vi "Test System.vi"() -> ()   [LabVIEW 2015]
uses:
  CAN Communication/Gas/Typedefs/Valves.ctl
  CAN Communication/Peltier/Typedefs/Peltier Temperature Sensors.ctl
  CAN Communication/Gas/Gas.lvclass
  Common/Buffers/Snapshot/Snapshot.lvclass
  CAN Communication/Peltier/Peltier.lvclass
panel:
  out "Status":string
  out "Temp":dbl caption="H2 Temp C" format="%#.2g"
  out "PPM":dbl caption="H2 PPM" format="%#.2g"
  in  "H2":bool
  out "Gas Board Errors":errorcluster
  out "Oil Present?":string
  in  "Oil Pres":bool
  out "Pelt":errorcluster caption="Peltier Board Errors"
  out "TS5":dbl caption="Temp Sensor 5" format="%#.2g"
  out "TS4":dbl caption="Temp Sensor 4" format="%#.2g"
  out "TS3":dbl caption="Temp Sensor 3" format="%#.2g"
  out "TS2":dbl caption="Temp Sensor 2" format="%#.2g"
  out "TS1":dbl caption="Temp Sensor 1" format="%#.2g"
  in  "Pelt":bool
  out "DAQ Errors":errorcluster
  out "Gas Pressure EX (PSI)":dbl format="%#.2g"
  in  "Valves":T1=52 items=["GV1"=33, "GV2"=34, "GV3"=35, "GV4"=36, "GV5"=37, "GV6"=38, "GV7"=39, "GV8"=40, "GV9"=41, "GV10"=42, "GV11"=43, "LV3"=51, "LV4"=52]
  out "Gas Pressure GC (PSI)":dbl format="%#.2g"
  in  "OK Button":bool
  out "Test Pressure (PSI)":dbl format="%#.2g"
  # "On Demand Information"
  # "Pressure Readings"
  # "Gas Board"
  # "Peltier Board"
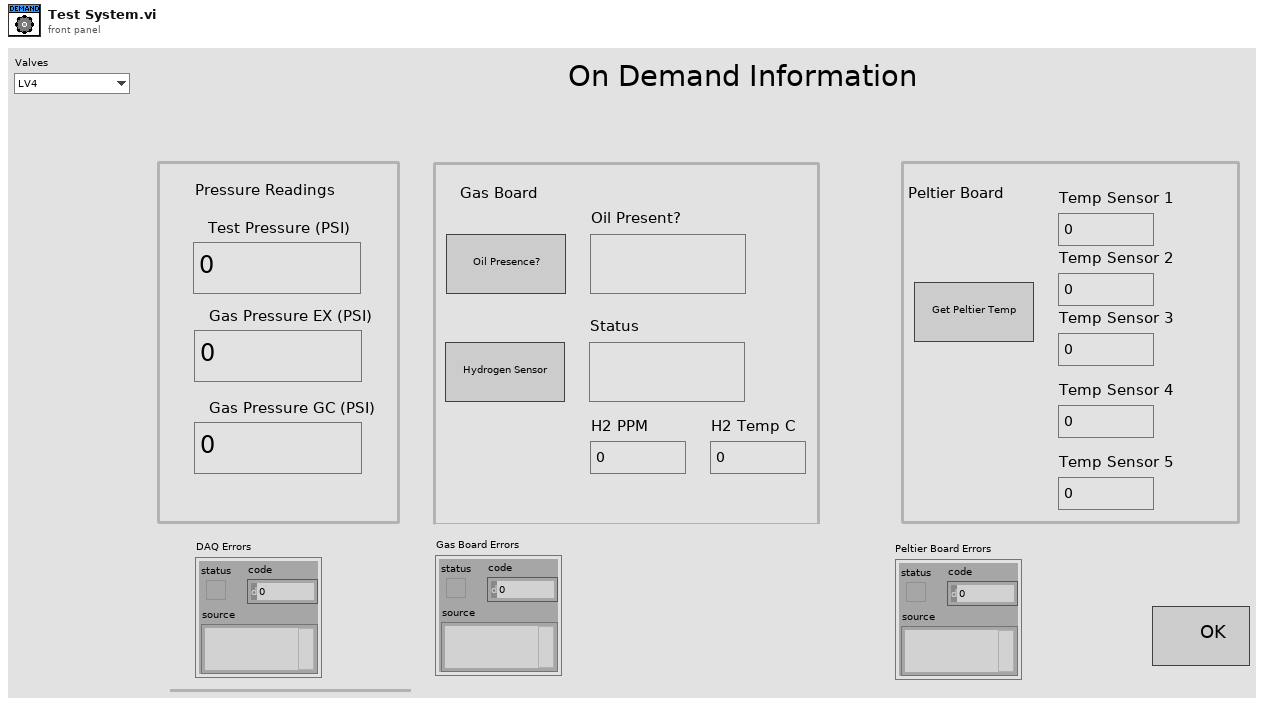
[diagram p1: front panel]
types:
  T1 = typedef "Gas.lvclass/Valves.ctl" = u16
  T2 = typedef "Gas.lvclass/Session Handle.ctl" = refnum<data-value>
  T3 = typedef "Snapshot.lvclass/Session Handle.ctl" = refnum<data-value>
  T4 = typedef "Peltier.lvclass/Peltier Temperature Sensors.ctl" = u16
  T5 = typedef "User Configuration.ctl" = cluster{"Password":string, "cDAQ Name":string, "CAN Interface":string}
  T6 = typedef "Peltier.lvclass/Session Handle.ctl" = refnum<data-value>
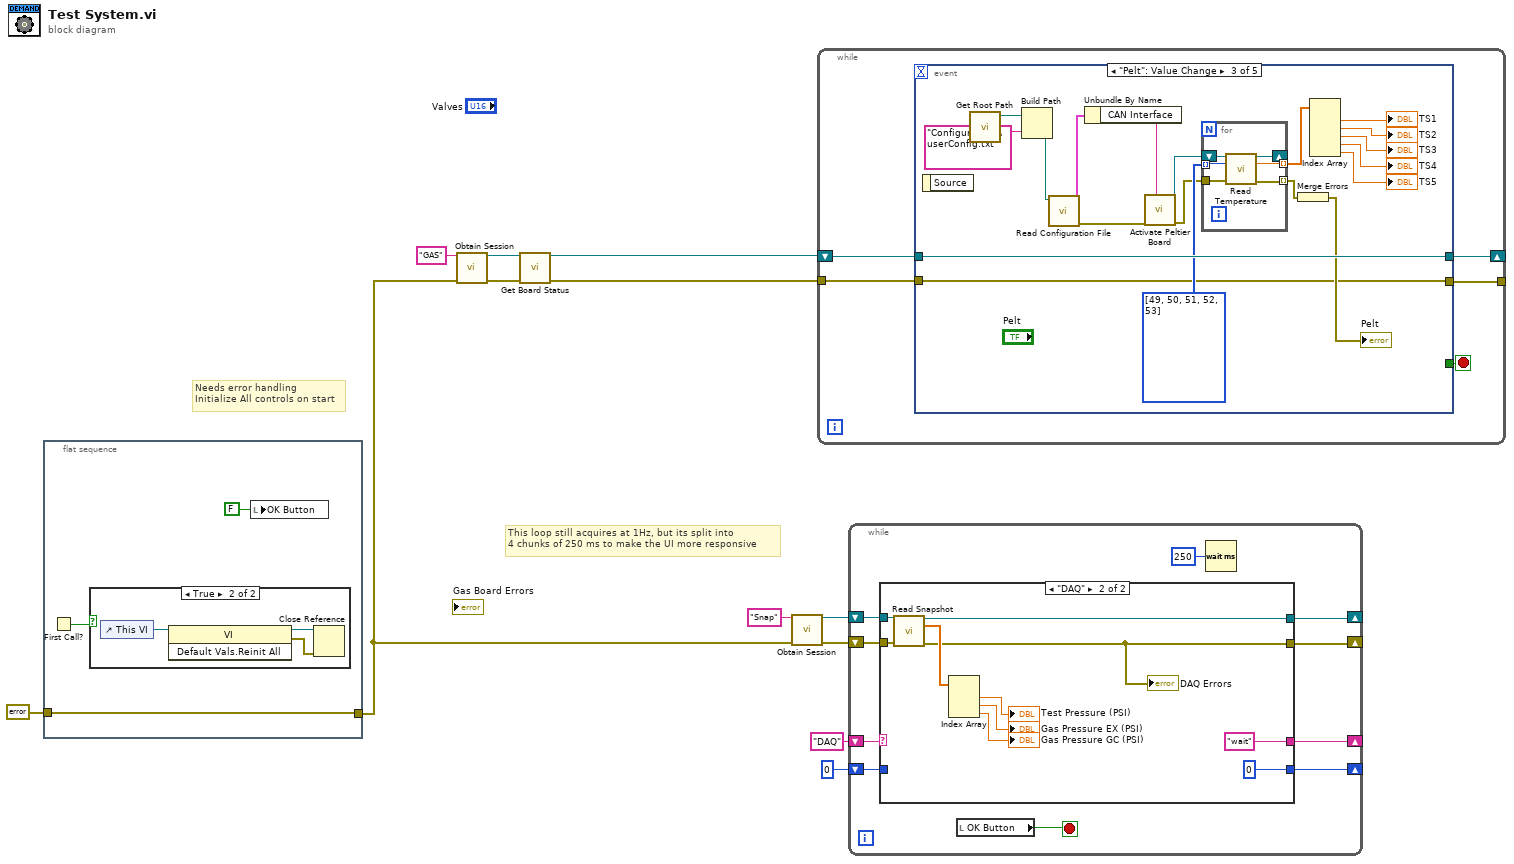
[diagram p0: block diagram]
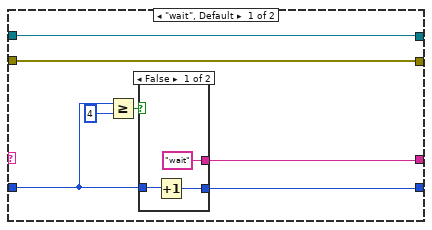
[diagram p2: hidden frame]
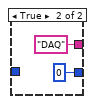
[diagram p3: hidden frame]
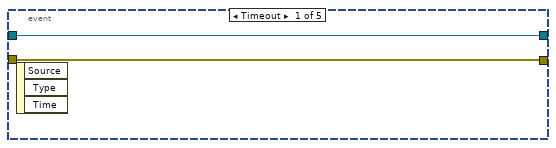
[diagram p5: hidden frame]
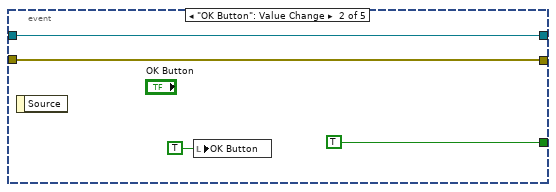
[diagram p6: hidden frame]
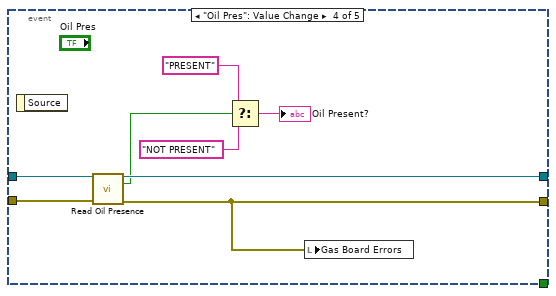
[diagram p7: hidden frame]
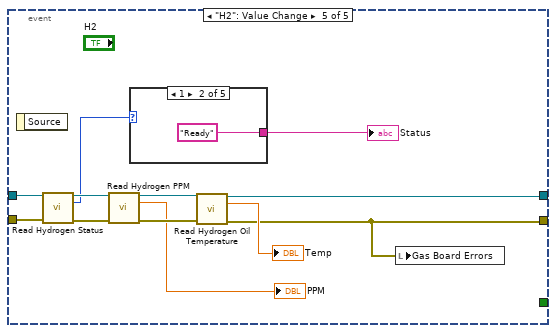
[diagram p8: hidden frame]
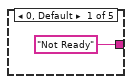
[diagram p9: hidden frame]
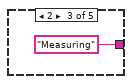
[diagram p10: hidden frame]
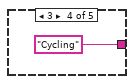
[diagram p11: hidden frame]
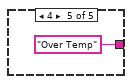
[diagram p12: hidden frame]
diagram:
  # "This loop still acquires at 1Hz, but its split into\n4 chunks of 250 ms to make the UI more responsive"
  # "Needs error handling\nInitialize All controls on start"
  n1 = flat-sequence {
    tunnel: errorcluster {"status"=FALSE, "code"=0, "source"=""} ("error in (no error)") -> [w14]
    tunnel: [w14] -> w1
    frame #0 {
      n2 = First Call?() -> (First Call?: T/F=w13:bool)
      n3 = case shown="True" w13 {
        frame False {
        }
        frame True {
          n4 = control-ref of="This VI"() -> (w18:refnum<vi>)
          n5 = invoke class="VI" method="Default Vals.Reinit All"(reference=w18) -> (reference out=w16:refnum<vi>, error out=w17:errorcluster)  [unwired: 2 in, 1 out]
          n6 = Close Reference(reference=w16, error in (no error)=w17) -> ()  [unwired: 1 out]
        }
      }
      n7 = local write "OK Button"(FALSE ("OK Button")) -> ()
    }
  }
  n8 = call "Obtain Session.vi"("Session  Name ()"="GAS", "error in (no error)"=w1) -> ("Session Handle"=w10:T2, "error out"=w9:errorcluster)  [unwired: 12 in]
  n9 = call "Get Board Status.vi"("Session Handle in"=w10, "error in (no error)"=w9) -> ("Session Handle out"=w8:T2, "error out"=w7:errorcluster)  [unwired: 11 in, 1 out]
  n10 = call "Obtain Session.vi"("Session  Name ()"="Snap", "error in (no error)"=w1) -> ("Session Handle"=w5:T3, "error out"=w4:errorcluster)  [unwired: 12 in]
  n11 = while {
    shift-right: [w21] -> _
    shift-left: w8 -> [w23]
    tunnel: w7 -> [w22]
    tunnel: [w20] -> _
    stop <- w19 stop-if-true
    n12 = event shown="[2] \"Pelt\": Value Change" {
      selector: _ -> [_ _ _ _ _]
      dyn-events: _ -> [_ _ _ _ _]
      timeout: _ -> [_ _ _ _ _]
      tunnel: w23 -> [w25 w29 w48 w61 w73]
      tunnel: w22 -> [w24 w28 w39 w62 w74]
      tunnel: [w25 w29 w48 w60 w67] -> w21
      tunnel: [w24 w28 w39 w55 w63] -> w20
      tunnel: [_ TRUE ("OK Button") _ _ _] -> w19
      event Timeout {
        n13 = event-data() -> ()  [unwired: 1 in, 3 out]
      }
      event "OK Button": Value Change {
        n14 = event-data() -> ()  [unwired: 1 in, 1 out]
        n15 = local write "OK Button"(TRUE ("OK Button")) -> ()
      }
      event "Pelt": Value Change {
        w47 = T4[] [49, 50, 51, 52, 53] items=["PTS1"=49, "PTS2"=50, "PTS3"=51, "PTS4"=52, "PTS5"=53, "PTS6"=54]
        n16 = event-data() -> ()  [unwired: 1 in, 1 out]
        n17 = call "Get Root Path.vi"() -> ("Root Path"=w35:path)  [unwired: 11 in]
        n18 = Build Path(base path=w35, name or relative path="Configuration\\userConfig.txt") -> (appended path=w37:path)
        n19 = call "Read Configuration File.vi"("Filepath"=w37) -> ("error out"=w36:errorcluster, "User Config"=w34:T5)  [unwired: 9 in]
        n20 = Unbundle By Name(w34) -> ("CAN Interface"=w33:string)
        n21 = call "Activate Peltier Board.vi"("CAN Interface"=w33, "error in (no error)"=w36) -> ("error out"=w32:errorcluster, "Session Handle Out"=w30:T6)  [unwired: 8 in]
        n22 = for {
          shift-right: [w53] -> _
          shift-left: w30 -> [w54]
          tunnel: [w52] -> w46 mode=indexing
          tunnel: w47 -> [w51] mode=indexing
          tunnel: w32 -> [w50]
          tunnel: [w49] -> w31 mode=indexing
          n23 = call "Read Temperature.vi"("Session Handle"=w54, "Pelt Temp Sensors"=w51, "error in (no error)"=w50) -> ("Session Handle Out"=w53:T6, "Temperature"=w52:dbl, "error out"=w49:errorcluster)  [unwired: 10 in]
        }
        n24 = Merge Errors(w31) -> (→"Pelt":errorcluster)
        n25 = Index Array(array=w46) -> (element #1=→"TS1":dbl, element #2=→"TS2":dbl, element #3=→"TS3":dbl, element #4=→"TS4":dbl, element #5=→"TS5":dbl)  [unwired: 5 in]
      }
      event "Oil Pres": Value Change {
        n26 = event-data() -> ()  [unwired: 1 in, 1 out]
        n27 = call "Read Oil Presence.vi"("Session Handle in"=w61, "error in (no error)"=w62) -> ("Session Handle out"=w60:T2, "Present?"=w56:bool, "error out"=w55:errorcluster)  [unwired: 11 in]
        n28 = Select(t="PRESENT", s=w56, f="NOT PRESENT") -> (s? t:f=→"Oil Present?":string)
        n29 = local write "Gas Board Errors"(w55) -> ()
      }
      event "H2": Value Change {
        n30 = event-data() -> ()  [unwired: 1 in, 1 out]
        n31 = call "Read Hydrogen Status.vi"("Session Handle in"=w73, "error in (no error)"=w74) -> ("Session Handle out"=w69:T2, "Status"=w64:u16, "error out"=w68:errorcluster)  [unwired: 8 in, 3 out]
        n32 = call "Read Hydrogen PPM.vi"("Session Handle in"=w69, "error in (no error)"=w68) -> ("Session Handle out"=w71:T2, "H2 PPM"=→"PPM":dbl, "error out"=w70:errorcluster)  [unwired: 10 in, 1 out]
        n33 = case shown="1" w64 {
          tunnel: ["Not Ready" "Ready" "Measuring" "Cycling" "Over Temp"] -> w72
          frame 0, Default {
          }
          frame 1 {
          }
          frame 2 {
          }
          frame 3 {
          }
          frame 4 {
          }
        }
        "Status" <- w72
        n34 = call "Read Hydrogen Oil Temperature.vi"("Session Handle in"=w71, "error in (no error)"=w70) -> ("Session Handle out"=w67:T2, "H2 Temp"=→"Temp":dbl, "error out"=w63:errorcluster)  [unwired: 10 in, 1 out]
        n35 = local write "Gas Board Errors"(w63) -> ()
      }
    }
  }
  n36 = while {
    shift-right: [w86] -> _
    shift-left: w5 -> [w87]
    shift-right: [w85] -> _
    shift-left: w4 -> [w88]
    shift-right: [w83] -> _
    shift-left: "DAQ" -> [w84]
    shift-right: [w82] -> _
    shift-left: 0 -> [w81]
    stop <- w89 stop-if-true
    n37 = case shown="\"DAQ\"" w84 {
      tunnel: w88 -> [w95 w111]
      tunnel: w87 -> [w96 w110]
      tunnel: [w96 w109] -> w86
      tunnel: [w95 w102] -> w85
      tunnel: [w90 "wait"] -> w83
      tunnel: [w91 0] -> w82
      tunnel: w81 -> [w92 _]
      frame "wait", Default {
        n38 = Greater Or Equal?(x=w92, y=4) -> (x >= y?=w93:bool)
        n39 = case shown="False" w93 {
          tunnel: w92 -> [w99 _]
          tunnel: [w98 0] -> w91
          tunnel: ["wait" "DAQ"] -> w90
          frame False {
            n40 = Increment(x=w99) -> (x+1=w98:i32)
          }
          frame True {
          }
        }
      }
      frame "DAQ" {
        n41 = call "Read Snapshot.vi"("Session Handle in"=w110, "error in (no error)"=w111) -> ("Session Handle out"=w109:T3, "Buffer"=w108:dbl[], "error out"=w102:errorcluster)  [unwired: 11 in]
        "DAQ Errors" <- w102
        n42 = Index Array(array=w108) -> (element #1=→"Test Pressure (PSI)":dbl, element #2=→"Gas Pressure EX (PSI)":dbl, element #3=→"Gas Pressure GC (PSI)":dbl)  [unwired: 3 in]
      }
    }
    n43 = local read "OK Button"() -> (w89:bool)
    n44 = Wait (ms)(milliseconds to wait=u32 250) -> ()  [unwired: 1 out]
  }
